vi "Config Data Type.vi"(8 "error in (no error)":errorcluster, 11 "GroupAbstract in":refnum<class "GroupAbstract.lvclass">) -> (0 "error out":errorcluster, 2 "Group Data Type":T1, 3 "GroupAbstract out":refnum<class "GroupAbstract.lvclass">)   [LabVIEW 2020, in "Vecto.lvlib" / "GroupAbstract.lvclass"]
uses:
  GroupAbstract.lvclass
  Group Data Type.ctl
  GroupAbstract.lvclass/GroupAbstract.ctl
  Group Config/Group Config.lvclass/Group Config.ctl
  Group Config/Group Config.lvclass
  Vecto.lvlib
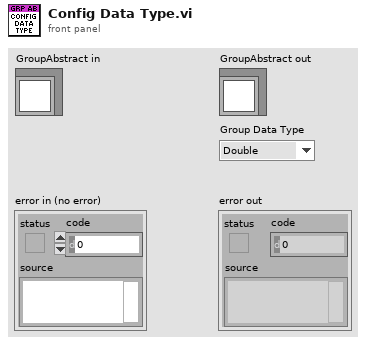
[diagram p1: front panel]
types:
  T1 = typedef "Vecto.lvlib/Group Data Type.ctl" = enum16{"Double", "String"}
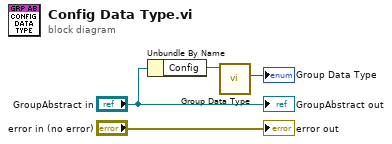
[diagram p0: block diagram]
diagram:
  n1 = Unbundle By Name("GroupAbstract in") -> ("Config"=w4:refnum<class "Group Config.lvclass">)
  n2 = call "Group Data Type.vi"("Group Config in"=w4) -> ("Data Type"=→"Group Data Type":T1)  [unwired: 8 in, 2 out]
  "error out" <- "error in (no error)"
  "GroupAbstract out" <- "GroupAbstract in"
